vi "read.vi"(8 "error in (no error)":errorcluster caption="错误输入（无错误）", 11 "TCP 输入":refnum<class "TCP.lvclass">) -> (0 "error out":errorcluster caption="错误输出", 2 "read":string, 3 "TCP 输出":refnum<class "TCP.lvclass">)   [LabVIEW 2016, in "中水三立SQL数据传输.lvlib" / "TCP.lvclass"]
uses:
  TCP.lvclass
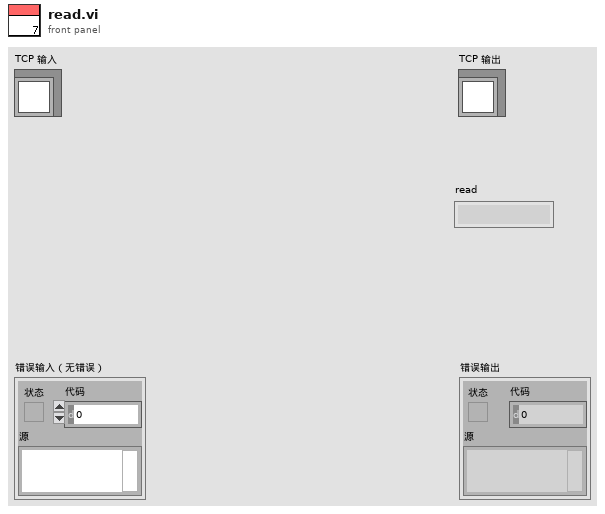
[diagram p1: front panel]
types:
  T1 = enum16{"Standard", "Buffered", "CRLF", "Immediate"}
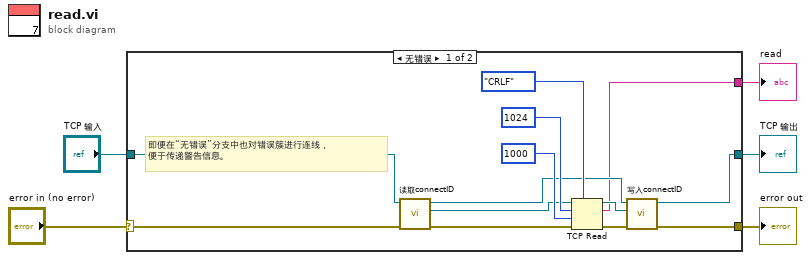
[diagram p0: block diagram]
diagram:
  n1 = case shown="无错误" "error in (no error)" {
    selector: "error in (no error)" -> [w8 w20]
    tunnel: [w9 w20] -> w1
    tunnel: [w11 w19] -> w3
    tunnel: "TCP 输入" -> [w15 w19]
    tunnel: [w6 _] -> w2
    frame No Error {
      # "即便在“无错误”分支中也对错误簇进行连线，\n便于传递警告信息。"
      n2 = call-dynamic "读取connectID.vi"("error in (no error)"=w8, "data_inter输入"=w15) -> ("error out"=w7:errorcluster, "connectID"=w14:refnum<k5>, "data_inter输出"=w12:refnum<class "TCP.lvclass">)  [unwired: 7 in]
      n3 = TCP Read(connection ID=w14, bytes to read=1024 ("读取的字节"), error in (no error)=w7, 7:T1."CRLF" ("模式（标准）"), 9:1000 ("超时毫秒(25000)")) -> (connection ID out=w13:refnum<k5>, data out=w6:string, error out=w10:errorcluster)
      n4 = call-dynamic "写入connectID.vi"("error in (no error)"=w10, "connectID"=w13, "data_inter输入"=w12) -> ("error out"=w9:errorcluster, "data_inter输出"=w11:refnum<class "TCP.lvclass">)  [unwired: 7 in]
    }
    frame Error {
    }
  }
  "error out" <- w1
  "TCP 输出" <- w3
  "read" <- w2
